vi "myRIO_BRig_Host_parse_dataTrial__readMain.vi"(0 "input_idxUnknown":i32, 1 "input_arrayUnknown":i32[][](array[numeric]), 2 "input_idxReward":i32, 3 "input_arrayReward":i32[][](array[numeric]), 4 "input_idxWrong":i32, 5 "input_arrayWrong":i32[][](array[numeric]), 6 "input_idxTimeout":i32, 7 "input_arrayTimeout":i32[][](array[numeric]), 10 "arrayIn_dataTrial":u16[][](array[numeric]), 12 "arrayIn_empty":i32[][](array[numeric])) -> (17 "output_countTrial":i32, 20 "output_idxUnknown":i32, 21 "output_arrayUnknown":i32[][](array[numeric]), 22 "output_idxReward":i32, 23 "output_arrayReward":i32[][](array[numeric]), 24 "output_idxWrong":i32, 25 "output_arrayWrong":i32[][](array[numeric]), 26 "output_idxTimeout":i32, 27 "output_arrayTimeout":i32[][](array[numeric]))   [LabVIEW 2014]
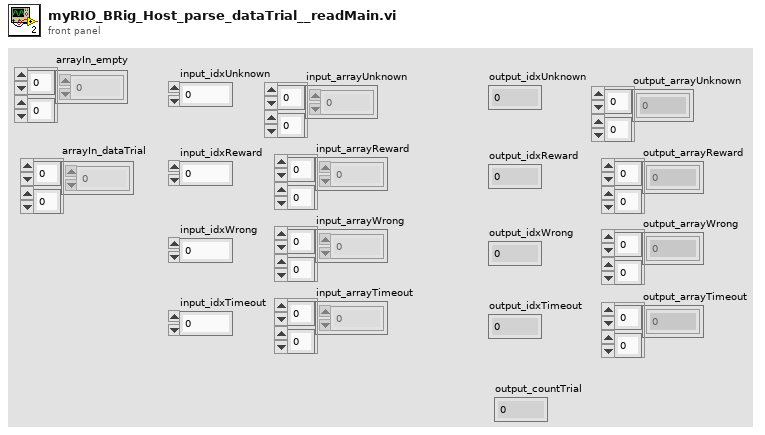
[diagram p1: front panel]
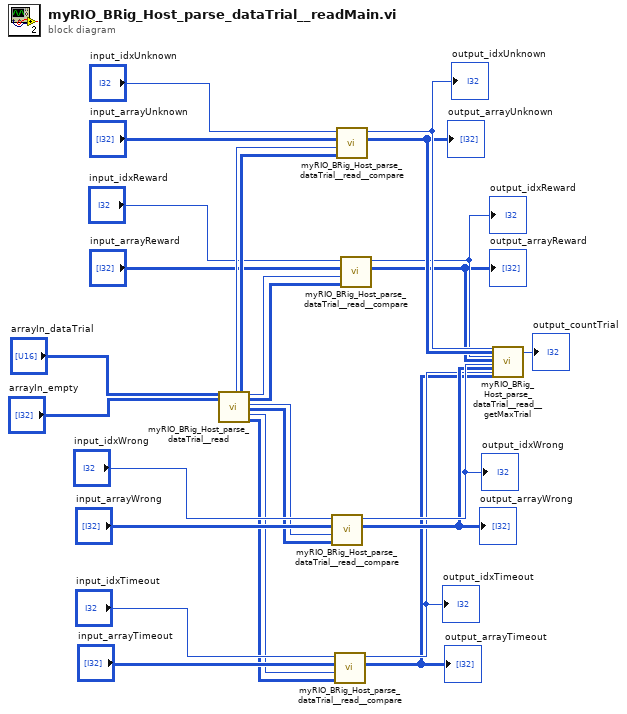
[diagram p0: block diagram]
diagram:
  n1 = call "myRIO_BRig_Host_parse_dataTrial__read.vi"("arrayIn_dataTrial"="arrayIn_dataTrial", "arrayIn_empty"="arrayIn_empty") -> ("output_idxUnknown"=w23:i32, "output_arrayUnknown"=w22:i32[][], "output_idxReward"=w19:i32, "output_arrayReward"=w18:i32[][], "output_idxWrong"=w15:i32, "output_arrayWrong"=w14:i32[][], "output_idxTimeout"=w11:i32, "output_arrayTimeout"=w10:i32[][])  [unwired: 10 in]
  n2 = call "myRIO_BRig_Host_parse_dataTrial__read__compare.vi"("input_arrayCtrl"=w14, "input_idxCtrl"=w15, "input_arraySample"="input_arrayWrong", "input_idxSample"="input_idxWrong") -> ("output_arraySample"=w4:i32[][], "output_idxSample"=w5:i32)  [unwired: 6 in]
  "output_idxWrong" <- w5
  "output_arrayWrong" <- w4
  n3 = call "myRIO_BRig_Host_parse_dataTrial__read__compare.vi"("input_arrayCtrl"=w10, "input_idxCtrl"=w11, "input_arraySample"="input_arrayTimeout", "input_idxSample"="input_idxTimeout") -> ("output_arraySample"=w2:i32[][], "output_idxSample"=w3:i32)  [unwired: 6 in]
  "output_idxTimeout" <- w3
  "output_arrayTimeout" <- w2
  n4 = call "myRIO_BRig_Host_parse_dataTrial__read__compare.vi"("input_arrayCtrl"=w22, "input_idxCtrl"=w23, "input_arraySample"="input_arrayUnknown", "input_idxSample"="input_idxUnknown") -> ("output_arraySample"=w8:i32[][], "output_idxSample"=w9:i32)  [unwired: 6 in]
  "output_idxUnknown" <- w9
  "output_arrayUnknown" <- w8
  n5 = call "myRIO_BRig_Host_parse_dataTrial__read__compare.vi"("input_arrayCtrl"=w18, "input_idxCtrl"=w19, "input_arraySample"="input_arrayReward", "input_idxSample"="input_idxReward") -> ("output_arraySample"=w6:i32[][], "output_idxSample"=w7:i32)  [unwired: 6 in]
  "output_idxReward" <- w7
  "output_arrayReward" <- w6
  n6 = call "myRIO_BRig_Host_parse_dataTrial__read__getMaxTrial.vi"("input_idxUnknown"=w9, "input_arrayUnknown"=w8, "input_idxReward"=w7, "input_arrayReward"=w6, "input_idxWrong"=w5, "input_arrayWrong"=w4, "input_idxTimeout"=w3, "input_arrayTimeout"=w2) -> ("output_maxTrial"=→"output_countTrial":i32)  [unwired: 19 in]
